vi "WPI_DMAAddChannelToStream_Counter.vi"(7 "CounterDevRef":T1={"DevStatus"={"status"=FALSE, "code"=0, "source"=""}, "CntIndex"=enum."Invalid"}, 8 "error in (no error)":errorcluster, 10 "Counter Output Type":enum16{"Counter Value", "Timer Value"}(ring), 11 "DMARef":T3) -> (0 "error out":errorcluster, 3 "DMARef":T3)   [LabVIEW 2017]
doc: "Specifies the data transferred in the DMA stream. Wire a device reference from the other WPI Robotics Library Open VIs to specify the data you want to receive. The order that the AddChannel VIs add data to the DMA stream defines the order that the Read VI returns the data.\n\nSpecifies the counter data transferred in the DMA stream.\n\nYou must open a reference to a DMA stream with the Open VI before using this VI.\n\nThis software is licensed. Open the labview\\readme\\WPI Robotics Library Open Source License.txt file for more information."
uses:
  <vilib>/Rock Robotics/WPI/DMA/WPI_DMARef.ctl
  <vilib>/Rock Robotics/WPI/Counter/WPI_CounterDevRef.ctl
  <vilib>/Rock Robotics/SystemInterfaces/Counter/FPGA_CounterCtrSystemIndex.ctl
  <vilib>/Rock Robotics/WPI/DMA/WPI_DMAChannelTypeEnum.ctl
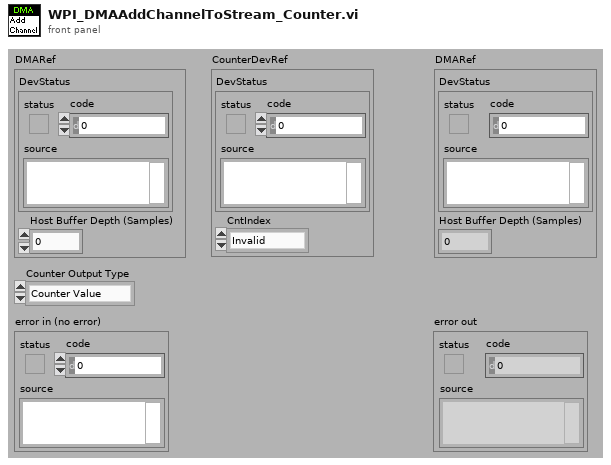
[diagram p1: front panel]
types:
  T1 = typedef "WPI_CounterDevRef.ctl" = cluster{"DevStatus":errorcluster, "CntIndex":T2}
  T2 = typedef "FPGA_CounterCtrSystemIndex.ctl" = enum8{"Ctr 0", "Ctr 1", "Ctr 2", "Ctr 3", "Ctr 4", "Ctr 5", "Ctr 6", "Ctr 7", "Invalid"}
  T3 = typedef "WPI_DMARef.ctl" = cluster{"DevStatus":errorcluster, "Host Buffer Depth (Samples)":u32}
  T4 = typedef "WPI_DMAChannelTypeEnum.ctl" = enum16{"AI (Raw)", "AI (Avg)", "Accumulator", "DI (Raw) Onboard", "DI (Filtered) Onboard", "DI (Raw) MXP", "DI (Filtered) MXP", "Analog Trigger", "Counter", "Counter (Timer)", "Encoder", "Encoder (Timer)", "Time Stamp"}
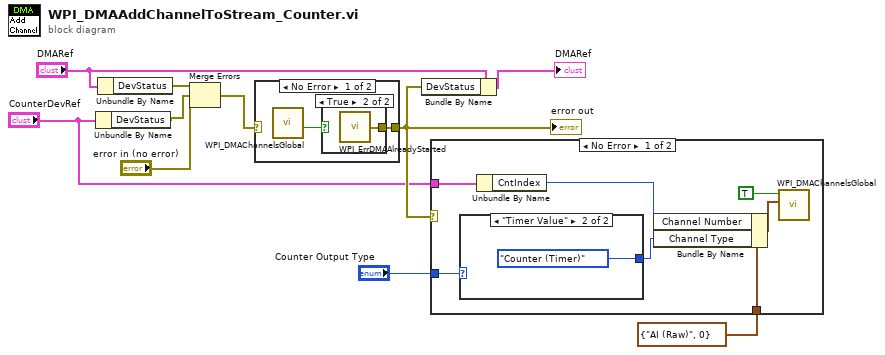
[diagram p0: block diagram]
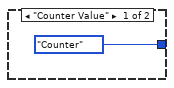
[diagram p2: hidden frame]
diagram:
  n1 = Unbundle By Name("CounterDevRef") -> ("DevStatus"=w3:errorcluster)
  n2 = Unbundle By Name("DMARef") -> ("DevStatus"=w4:errorcluster)
  n3 = Merge Errors(w4, w3, "error in (no error)") -> (w1:errorcluster)
  n4 = case shown="No Error" w1 {
    selector: w1 -> [_ w14]
    tunnel: [w11 w14] -> w9
    frame No Error {
      n5 = call <vilib>:"WPI_DMAChannelsGlobal.vi"() -> ("Started"=w12:bool)  [unwired: 4 in, 7 out]
      n6 = case shown="True" w12 {
        tunnel: [_ w13] -> w11
        frame False {
        }
        frame True {
          n7 = call <vilib>:"WPI_ErrDMAAlreadyStarted.vi"() -> ("error out"=w13:errorcluster)
        }
      }
    }
    frame Error {
    }
  }
  "error out" <- w9
  n8 = Bundle By Name(cluster="DMARef", "DevStatus"=w9) -> (→"DMARef":T3)
  n9 = case shown="No Error" w9 {
    tunnel: "CounterDevRef" -> [w20 _]
    tunnel: cluster{"Channel Type":T4, "Channel Number":u8} {"Channel Type"=enum."AI (Raw)", "Channel Number"=0} ("Channel") -> [w19 _]
    tunnel: "Counter Output Type" -> [w15 _]
    frame No Error {
      n10 = case shown="\"Timer Value\"" w15 {
        tunnel: [WPI_DMAChannelTypeEnum."Counter" ("Channel Type") WPI_DMAChannelTypeEnum."Counter (Timer)" ("Channel Type")] -> w17
        frame "Counter Value" {
        }
        frame "Timer Value" {
        }
      }
      n11 = Unbundle By Name(w20) -> ("CntIndex"=w16:T2)
      n12 = Bundle By Name(cluster=w19, "Channel Number"=w16, "Channel Type"=w17) -> (w18:cluster{"Channel Type":T4, "Channel Number":u8})
      n13 = call <vilib>:"WPI_DMAChannelsGlobal.vi"("Channel"=w18, "Add"=TRUE) -> ()  [unwired: 2 in, 8 out]
    }
    frame Error {
    }
  }
